vi "BNC505.vi"() -> ()   [LabVIEW 2013]
panel:
  in  "Pressure reading (mA)":string
  in  "Pressure reading (bara)":string
  in  "Pulse Duration fs":string
  in  "Path to Folder":path
  in  "Comments":string
  in  "FLSH":bool
  in  "SEND":bool
  out "error out":errorcluster
  in  "stop":bool
  out "read buffer":string
  in  "error in (no error)":errorcluster
  in  "VISA resource name":refnum<visa-resource-name>
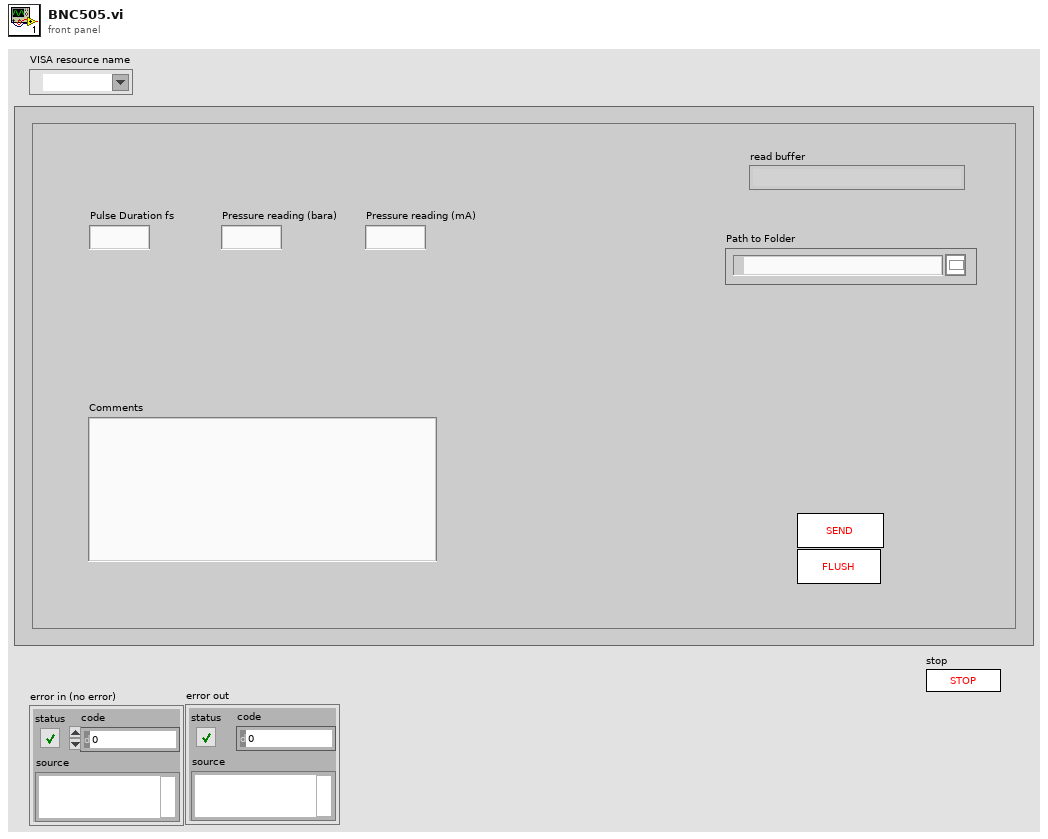
[diagram p1: front panel]
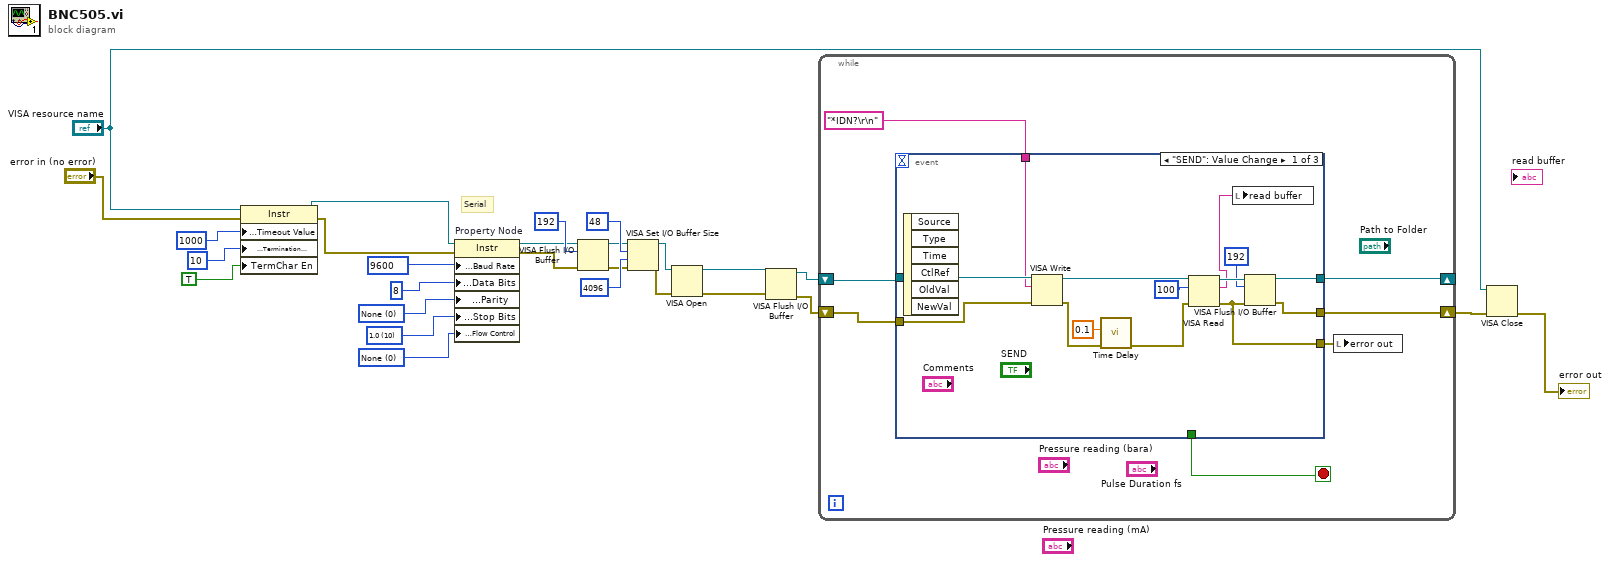
[diagram p0: block diagram]
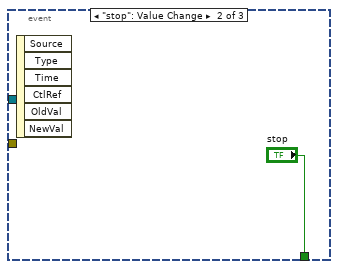
[diagram p2: hidden frame]
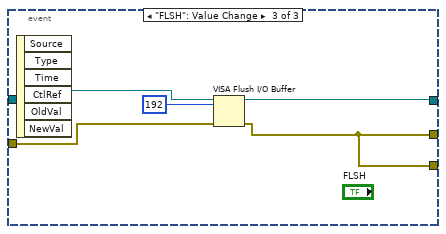
[diagram p3: hidden frame]
diagram:
  w7 = u32 9600 items=["4800"=4600, "9600"=9600, "19200"=19200, "38400"=38400, "57600"=57600, "115200"=115200] ("Baud Rate (make sure matches instrument)")
  w4 = u16 0 items=["None"=0, "XON/XOFF"=1, "RTS/CTS"=2, "DTR/DSR"=4] ("Serial Settings:Serial Flow Control")
  w15 = u16 10 items=["1.0"=10, "1.5"=15, "2.0"=20] ("Serial Settings:Serial Stop Bits")
  w16 = u16 0 items=["None", "Odd", "Even", "Mark", "Space"] ("Serial Settings:Serial Parity")
  # "Serial"
  n1 = property class="Instr"(reference="VISA resource name", error in="error in (no error)", "General Settings:Timeout Value"=u32 1000, "Message Based Settings:Termination Character"=u8 10, "TermChar En"=TRUE ("Message Based Settings:Termination Character Enable")) -> (reference out=w5:refnum<visa-resource-name>, error out=w6:errorcluster)
  n2 = property on="Property Node" class="Instr"(reference=w5, error in=w6, "Serial Settings:Baud Rate"=w7, "Serial Settings:Data Bits"=u16 8 ("Serial Settings:Serial Data Bits"), "Serial Settings:Parity"=w16, "Serial Settings:Stop Bits"=w15, "Serial Settings:Flow Control"=w4) -> (reference out=w9:refnum<visa-resource-name>, error out=w8:errorcluster)
  n3 = VISA Flush I/O Buffer(VISA resource name=w9, mask (16)=u16 192, error in (no error)=w8) -> (VISA resource name out=w10:refnum<visa-resource-name>, error out=w11:errorcluster)
  n4 = VISA Set I/O Buffer Size(VISA resource name=w10, mask (16)=u16 48, size (4096)=u32 4096 ("size (0)"), error in (no error)=w11) -> (VISA resource name out=w3:refnum<visa-resource-name>, error out=w2:errorcluster)
  n5 = VISA Open(error in (no error)=w2, VISA resource name=w3) -> (VISA resource name=w25:refnum<visa-resource-name>, error out=w24:errorcluster)  [unwired: 3 in]
  n6 = VISA Flush I/O Buffer(VISA resource name=w25, error in (no error)=w24) -> (VISA resource name out=w22:refnum<visa-resource-name>, error out=w23:errorcluster)  [unwired: 1 in]
  n7 = while {
    shift-right: [w29] -> _
    shift-left: w22 -> [w34]
    shift-right: [w32] -> w27
    shift-left: w23 -> [w30]
    stop <- w33 stop-if-true
    n8 = event shown="[0] \"SEND\": Value Change" {
      selector: _ -> [_ _ _]
      dyn-events: _ -> [_ _ _]
      timeout: _ -> [_ _ _]
      tunnel: w34 -> [w38 _ w52]
      tunnel: [_ "stop" _] -> w33
      tunnel: [w46 _ w50] -> w32
      tunnel: [w45 _ w51] -> w29
      tunnel: [w43 _ w50] -> w31
      tunnel: w30 -> [w37 _ w54]
      tunnel: "*IDN?\r\n" ("string") -> [w35 _ _]
      event "SEND": Value Change {
        n9 = event-data() -> ()  [unwired: 1 in, 6 out]
        n10 = VISA Write(VISA resource name=w38, write buffer=w35, error in (no error)=w37) -> (VISA resource name out=w48:refnum<visa-resource-name>, error out=w41:errorcluster)  [unwired: 1 out]
        n11 = call "Time Delay"("error in (no error)"=w41, "Delay Time (s)"=0.1) -> ("error out"=w40:errorcluster)  [unwired: 9 out]
        n12 = VISA Read(VISA resource name=w48, byte count=u32 100, error in (no error)=w40) -> (VISA resource name out=w44:refnum<visa-resource-name>, read buffer=w36:string, error out=w43:errorcluster)  [unwired: 1 out]
        n13 = local write "read buffer"(w36) -> ()
        n14 = VISA Flush I/O Buffer(VISA resource name=w44, mask (16)=u16 192, error in (no error)=w43) -> (VISA resource name out=w45:refnum<visa-resource-name>, error out=w46:errorcluster)
      }
      event "stop": Value Change {
        n15 = event-data() -> ()  [unwired: 1 in, 6 out]
      }
      event "FLSH": Value Change {
        n16 = event-data() -> ()  [unwired: 1 in, 6 out]
        n17 = VISA Flush I/O Buffer(VISA resource name=w52, mask (16)=u16 192, error in (no error)=w54) -> (VISA resource name out=w51:refnum<visa-resource-name>, error out=w50:errorcluster)
      }
    }
    n18 = local write "error out"(w31) -> ()
  }
  n19 = VISA Close(VISA resource name="VISA resource name", error in (no error)=w27) -> (error out=→"error out":errorcluster)
